vi "Facade.vi"(0 "Data In":T4 caption="数据输入", 2 "Display State In":T2 caption="显示状态输入", 3 "Container State":T3 caption="容器状态") -> (6 "Data Out":T4 caption="数据输出", 7 "Display State Out":T2 caption="显示状态输出", 8 "Action":T1 caption="动作")   [LabVIEW 2016, in "ArrayTree.xctl"]
uses:
  ArrayTree.xctl
  Data.ctl
  <vilib>/_xctls/Container State.ctl
  Status.ctl
  <vilib>/_xctls/Action.ctl
  <vilib>/_xctls/XControlSupport.lvlib
panel:
  in  "树形":string(tree)
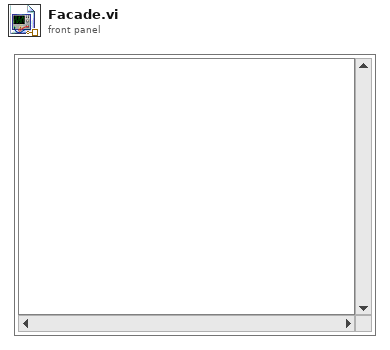
[diagram p1: front panel]
types:
  T1 = typedef "XControlSupport.lvlib/Action.ctl" = cluster{"Data Changed?":bool, "State Changed?":bool, "Action Name":string}
  T2 = typedef "ArrayTree.xctl/Status.ctl" = cluster{"TopLevelItemName":string, "ChildItemArr":cluster{"ChildDimName":string, "ChildDimSize":u64}[]}[]
  T3 = typedef "XControlSupport.lvlib/Container State.ctl" = cluster{"Indicator?":bool, "Run Mode?":bool, " Refnum":refnum<vi>}
  T4 = typedef "ArrayTree.xctl/Data.ctl" = cluster{"TopLevelItemName":string, "ChildItemArr":cluster{"ChildDimName":string, "ChildDimSize":u64}[]}[]
  T5 = cluster{"ChildDimName":string, "ChildDimSize":u64}[]
  T6 = cluster{"ChildDimName":string, "ChildDimSize":u64}
  T7 = cluster{"TopLevelItemName":string, "ChildItemArr":cluster{"ChildDimName":string, "ChildDimSize":u64}[]}
  T8 = cluster{"TopLevelItemName":string, "ChildItemArr":cluster{"ChildDimName":string, "ChildDimSize":u64}[]}[]
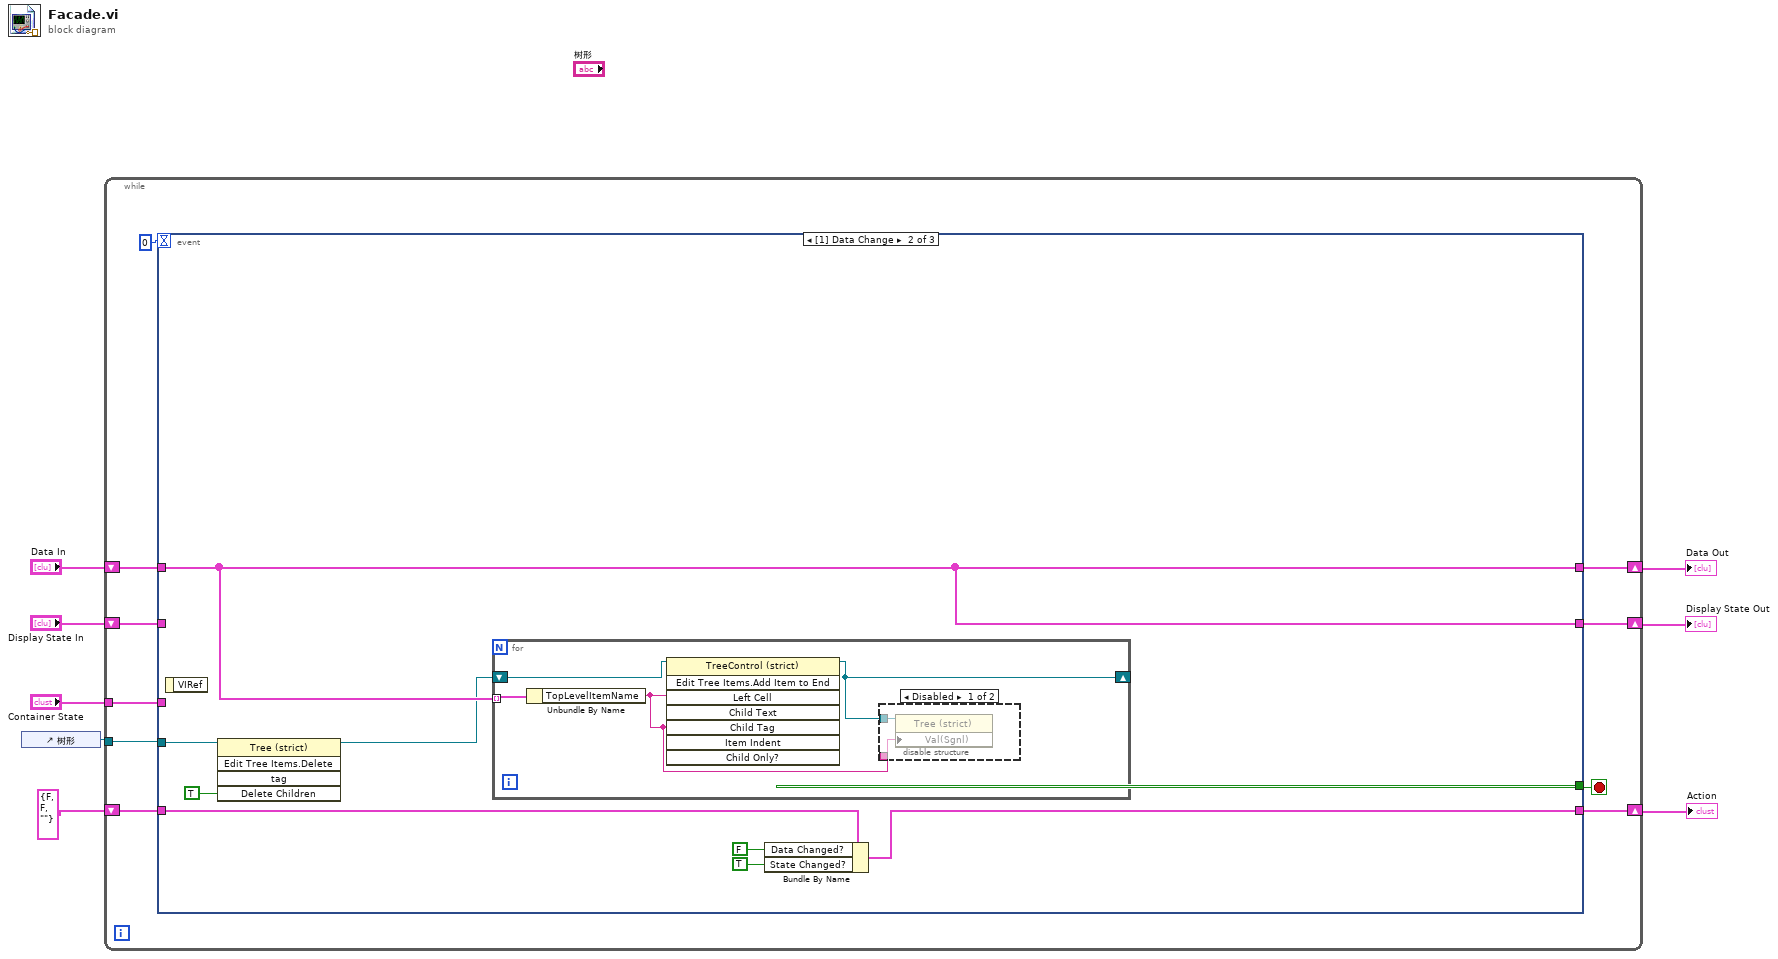
[diagram p0: block diagram]
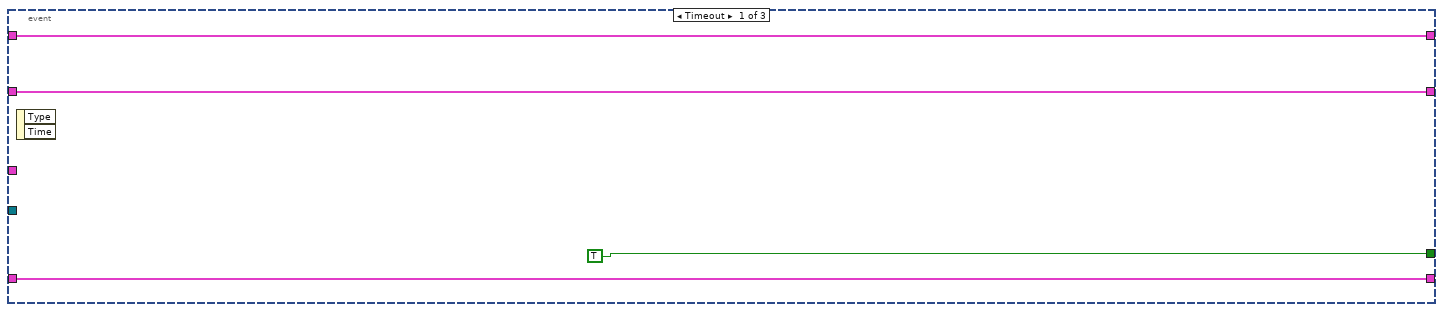
[diagram p2: hidden frame]
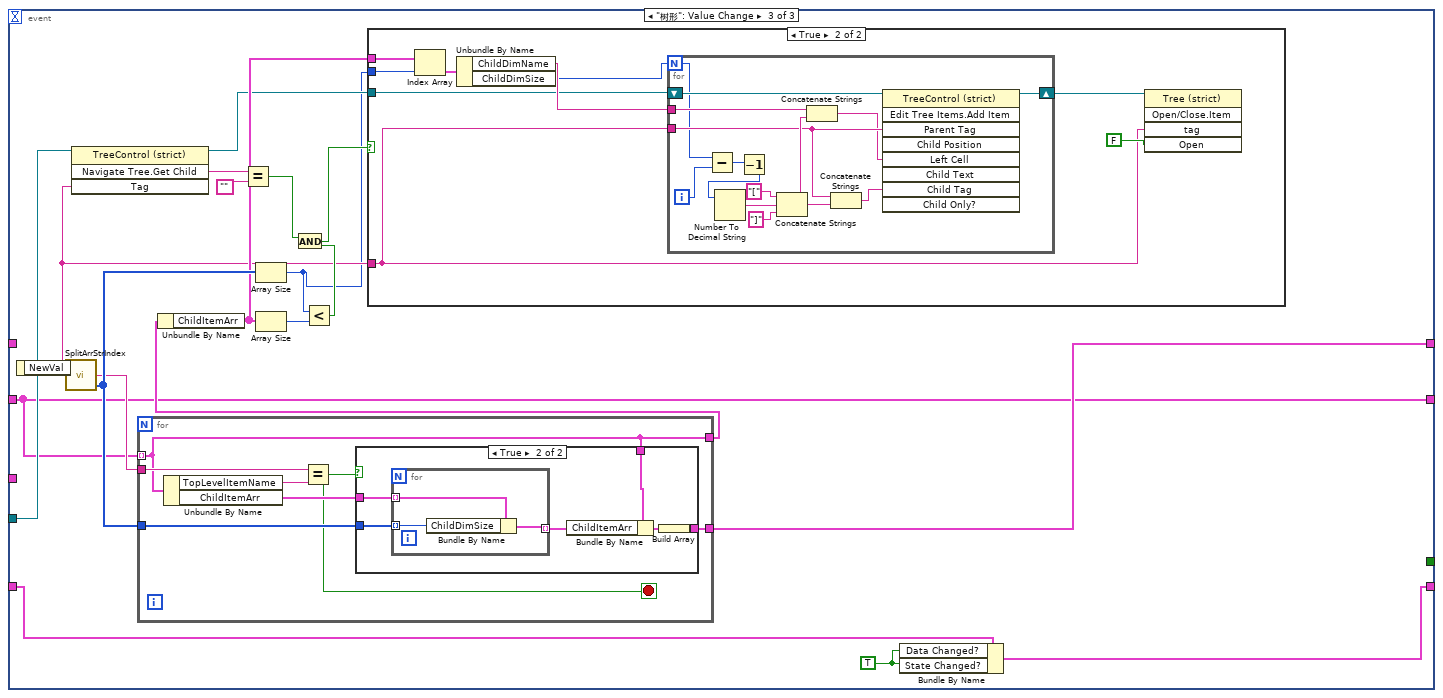
[diagram p4: hidden frame]
diagram:
  n1 = control-ref of="树形"() -> (w1:refnum<vi>)
  n2 = while {
    shift-right: [w17] -> w5
    shift-left: "Display State In" -> [w18]
    tunnel: "Container State" -> [w14]
    shift-right: [w12] -> w8
    shift-left: "Data In" -> [w13]
    shift-right: [w10] -> w3
    shift-left: T1 {"Data Changed?"=FALSE, "State Changed?"=FALSE, "Action Name"=""} ("Action") -> [w11]
    tunnel: w1 -> [w9]
    stop <- w16 stop-if-true
    n3 = event shown="[1] Data Change" {
      selector: _ -> [_ _ _]
      dyn-events: _ -> [_ _ _]
      timeout: 0 -> [_ _ _]
      tunnel: w18 -> [w20 _ w40]
      tunnel: [w20 w30 w40] -> w17
      tunnel: [TRUE _ _] -> w16
      tunnel: w14 -> [_ _ _]
      tunnel: w13 -> [w19 w30 _]
      tunnel: [w19 w30 w55] -> w12
      tunnel: [w21 w25 w39] -> w10
      tunnel: w11 -> [w21 w26 w37]
      tunnel: w9 -> [_ w28 w46]
      event Timeout {
        n4 = event-data() -> ()  [unwired: 3 out]
      }
      event Data Change {
        n5 = event-data() -> ()  [unwired: 2 out]
        n6 = invoke class="Tree (strict)" method="Edit Tree Items.Delete"(reference=w28, "Delete Children"=TRUE ("删除子项？")) -> (reference out=w27:refnum<vi>)  [unwired: 3 in, 4 out]
        n7 = for {
          tunnel: w30 -> [w33] mode=indexing
          shift-right: [w31] -> _
          shift-left: w27 -> [w34]
          n8 = Unbundle By Name(w33) -> ("TopLevelItemName"=w32:string)
          n9 = invoke class="TreeControl (strict)" method="Edit Tree Items.Add Item to End"(reference=w34, "Left Cell"=w32, "Child Tag"=w32) -> (reference out=w31:refnum<vi>)  [unwired: 5 in, 7 out]
          n10 = disable-structure shown="Disabled" {
            disable-tunnel: w32 -> [w36 _]
            disable-tunnel: w31 -> [w35 _]
            frame Disabled {
              n11 = property class="Tree (strict)"(reference=w35, "Val(Sgnl)"=w36) -> ()  [unwired: 1 in, 2 out]
            }
            frame Enabled {
            }
          }
        }
        n12 = Bundle By Name(cluster=w26, "Data Changed?"=FALSE, "State Changed?"=TRUE) -> (w25:T1)
      }
      event "树形": Value Change {
        w38 = TRUE ("State Changed?")
        n13 = event-data() -> ("NewVal"=w42:string)  [unwired: 1 out]
        n14 = call "SplitArrStrIndex.vi"("ArrayStr"=w42) -> ("ArrayIndex"=w53:u64[], "ArrayName"=w43:string)  [unwired: 3 out]
        n15 = invoke class="TreeControl (strict)" method="Navigate Tree.Get Child"(reference=w46, "Tag"=w42) -> (reference out=w45:refnum<vi>, "Navigate Tree:Get Child"=w50:string)  [unwired: 2 in, 2 out]
        n16 = for {
          tunnel: w40 -> [w79] mode=indexing
          tunnel: w43 -> [w81]
          tunnel: w53 -> [w84]
          tunnel: [w83] -> w55
          tunnel: [w79] -> w54
          stop <- w80 stop-if-true
          n17 = Unbundle By Name(w79) -> ("TopLevelItemName"=w82:string, "ChildItemArr"=w85:T5)
          n18 = Equal?(x=w81, y=w82) -> (x = y?=w80:bool)
          n19 = case shown="True" w80 {
            tunnel: w79 -> [_ w91]
            tunnel: w85 -> [_ w90]
            tunnel: w84 -> [_ w89]
            tunnel: [_ w86] -> w83
            frame False {
            }
            frame True {
              n20 = for {
                tunnel: w90 -> [w93] mode=indexing
                tunnel: w89 -> [w94] mode=indexing
                tunnel: [w92] -> w88 mode=indexing
                n21 = Bundle By Name(cluster=w93, "ChildDimSize"=w94) -> (w92:T6)
              }
              n22 = Bundle By Name(cluster=w91, "ChildItemArr"=w88) -> (w87:T7)
              n23 = Build Array(w87) -> (w86:T8)
            }
          }
        }
        n24 = Unbundle By Name(w54) -> ("ChildItemArr"=w52:T5)
        n25 = Equal?(x=w50, y="") -> (x = y?=w44:bool)
        n26 = Array Size(array=w53) -> (size(s)=w41:i32)
        n27 = Array Size(array=w52) -> (size(s)=w51:i32)
        n28 = Less?(x=w41, y=w51) -> (x < y?=w48:bool)
        n29 = And(x=w44, y=w48) -> (x .and. y?=w47:bool)
        n30 = case shown="True" w47 {
          tunnel: w52 -> [_ w64]
          tunnel: w41 -> [_ w60]
          tunnel: w45 -> [_ w58]
          tunnel: w42 -> [_ w57]
          frame False {
          }
          frame True {
            n31 = Index Array(array=w64, index=w60) -> (element=w61:T6)
            n32 = Unbundle By Name(w61) -> ("ChildDimName"=w63:string, "ChildDimSize"=w56:u64)
            n33 = for {
              N: w56 -> [w70]
              tunnel: w63 -> [w75]
              tunnel: w57 -> [w72]
              shift-right: [w65] -> w59
              shift-left: w58 -> [w73]
              i -> [w69]
              n34 = Subtract(x=w70, y=w69) -> (x-y=w68:i32)
              n35 = Decrement(x=w68) -> (x-1=w67:i32)
              n36 = Number To Decimal String(number=w67) -> (decimal integer string=w78:string)  [unwired: 1 out]
              n37 = Concatenate Strings("[" ("字符串"), w78, "]" ("字符串")) -> (w74:string)
              n38 = Concatenate Strings(w75, w74) -> (w71:string)
              n39 = Concatenate Strings(w72, w74) -> (w66:string)
              n40 = invoke class="TreeControl (strict)" method="Edit Tree Items.Add Item"(reference=w73, "Parent Tag"=w72, "Left Cell"=w71, "Child Tag"=w66) -> (reference out=w65:refnum<vi>)  [unwired: 5 in, 8 out]
            }
            n41 = invoke class="Tree (strict)" method="Open/Close.Item"(reference=w59, "tag"=w57, "Open"=FALSE ("打开？")) -> ()  [unwired: 2 in, 5 out]
          }
        }
        n42 = Bundle By Name(cluster=w37, "Data Changed?"=w38, "State Changed?"=w38) -> (w39:T1)
      }
    }
  }
  "Display State Out" <- w5
  "Data Out" <- w8
  "Action" <- w3
